vi "New JSON (Boolean).vi"(8 "error in (no error)":errorcluster, 10 "value":bool) -> (0 "error out":errorcluster, 3 "JSON Value out":refnum<class "JSON Value.lvclass">)   [LabVIEW 2016, in "JSON Value.lvclass"]
doc: "Creates a new JSON Boolean initialized with the given value"
uses:
  JSON Value.lvclass
  JSON Types.ctl
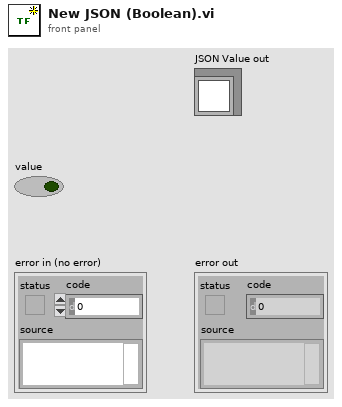
[diagram p1: front panel]
types:
  T1 = typedef "JSON Value.lvclass/JSON Types.ctl" = enum8{"String", "Numeric", "Boolean", "NULL", "Object", "Array"}
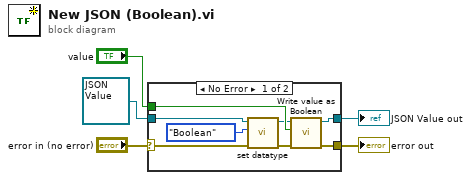
[diagram p0: block diagram]
diagram:
  n1 = case shown="No Error" "error in (no error)" {
    selector: "error in (no error)" -> [w11 w15]
    tunnel: [w12 w15] -> w4
    tunnel: [w13 w14] -> w3
    tunnel: refnum<class "JSON Value.lvclass"> refnum ("JSON out") -> [w8 w14]
    tunnel: "value" -> [w10 _]
    frame No Error {
      n2 = call "set datatype.vi"("error in (no error)"=w11, "datatype"=JSON_Types."Boolean", "JSON Helper in"=w8) -> ("error out"=w9:errorcluster, "JSON Helper out"=w7:refnum<class "JSON Value.lvclass">)  [unwired: 7 in]
      n3 = call "Write value as Boolean.vi"("error in (no error)"=w9, "value"=w10, "JSON Value in"=w7) -> ("error out"=w12:errorcluster, "JSON Value out"=w13:refnum<class "JSON Value.lvclass">)  [unwired: 7 in]
    }
    frame Error {
    }
  }
  "error out" <- w4
  "JSON Value out" <- w3
